vi "extract deleted files.vi"(1 "Input Array":path[][](array[path])) -> (0 "Deleted Files":path[](array[path]))   [LabVIEW 2011]
doc: "This VI is necessary to remove the <Not A Path> results from the Input Array so that only the deleted Files are reported."
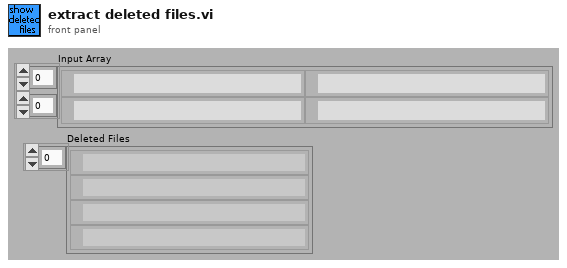
[diagram p1: front panel]
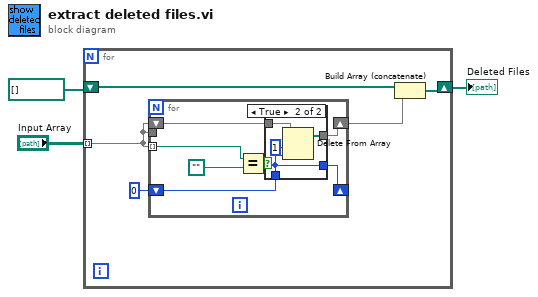
[diagram p0: block diagram]
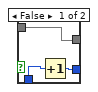
[diagram p2: hidden frame]
diagram:
  n1 = for {
    tunnel: "Input Array" -> [w7] mode=indexing
    shift-right: [w5] -> w1
    shift-left: path[] [] ("Array") -> [w6]
    n2 = for {
      tunnel: w7 -> [_]
      tunnel: w7 -> [w14] mode=indexing
      shift-right: [w13] -> w4
      shift-left: w7 -> [w12]
      shift-right: [w10] -> _
      shift-left: 0 -> [w11]
      n3 = Equal?(x=w14, y=path "") -> (x = y?=w15:bool)
      n4 = case shown="True" w15 {
        tunnel: [w18 w21] -> w13
        tunnel: w12 -> [w18 w20]
        tunnel: w11 -> [w16 w19]
        tunnel: [w17 w19] -> w10
        frame False {
          n5 = Increment(x=w16) -> (x+1=w17:i32)
        }
        frame True {
          n6 = Delete From Array(array=w20, length=1 ("Length"), index=w19) -> (array with subset deleted=w21:path[])  [unwired: 1 out]
        }
      }
    }
    n7 = Build Array (concatenate)(w6, w4) -> (w5:path[])
  }
  "Deleted Files" <- w1
